vi "observacao.vi"() -> ()   [LabVIEW 2018, in "Shared_160.lvlib"] (continued)
              tunnel: [w1811 w1813] -> w1790
              tunnel: [w1811 w1814] -> w1789
              tunnel: w1788 -> [_ w1814]
              tunnel: w1787 -> [_ w1813]
              frame False {
                w1811 = 0.0 ("DeslocRA")
                n1518 = property on="Calagem" class="Bool"("Disabled"=u8 2) -> ()  [unwired: 2 in, 2 out]
              }
              frame True {
                n1519 = property on="Calagem" class="Bool"("Disabled"=u8 0) -> ()  [unwired: 2 in, 2 out]
              }
            }
            "DeslocRA" <- w1789
            "DeslocDEC" <- w1790
          }
          frame "GUIDER" {
            w1959 = 1 ("lower limit")
            w1960 = 400 ("upper limit")
            # "PROCESSO VARIABLE TRACKING"
            n1520 = Not(x="ExternalTracking") -> (.not. x?=w1945:bool)
            n1521 = call "Borda Subida.vi"("Entrada"="VARIABLE \nTRACKING") -> ("Boolean"=w1947:bool)  [unwired: 4 in]
            n1522 = call "Borda.vi"("Entrada"="VARIABLE \nTRACKING") -> ("Boolean"=w1948:bool)  [unwired: 4 in]
            n1523 = And(x=w1945, y=w1947) -> (x .and. y?=w1946:bool)
            n1524 = case shown="True" w1948 {
              frame False {
              }
              frame True {
                w2017 = "0" ("Set Point")
                w2023 = u16 2 items=["ZERO", "AH", "DEC", "TUBO", "CUP"] ("Controlador")
                w2020 = u16 1 items=["ZERO", "AH", "DEC", "TUBO", "CUP"] ("Controlador")
                # "Enviando ZERO o controlador para o movimento"
                n1525 = call "Monta Comando.vi"("Set Point"=w2017, "Comando"="GIRAR_VEL", "Dispositivo"="EIXO" ("Comando"), "Controlador"=w2020) -> ()  [unwired: 1 in, 5 out]
                n1526 = call "Monta Comando.vi"("Set Point"=w2017, "Comando"="GIRAR_VEL", "Dispositivo"="EIXO" ("Comando"), "Controlador"=w2023) -> ()  [unwired: 1 in, 5 out]
              }
            }
            n1527 = case shown="True" w1946 {
              frame False {
              }
              frame True {
                w2034 = u16 2 items=["ZERO", "AH", "DEC", "TUBO", "CUP"] ("Controlador")
                w2031 = u16 1 items=["ZERO", "AH", "DEC", "TUBO", "CUP"] ("Controlador")
                # "Enviar esses Valores \npara os controladores"
                n1528 = property on="Calagem" class="Bool"("Disabled"=u8 2) -> ()  [unwired: 2 in, 2 out]
                n1529 = Number To Decimal String(number="RA  RATE") -> (decimal integer string=w2027:string)  [unwired: 1 in]
                n1530 = Number To Decimal String(number="DEC RATE") -> (decimal integer string=w2025:string)  [unwired: 1 in]
                n1531 = call "Monta Comando.vi"("Set Point"=w2027, "Comando"="GIRAR_VEL", "Dispositivo"="EIXO" ("Comando"), "Controlador"=w2031) -> ()  [unwired: 1 in, 5 out]
                n1532 = call "Monta Comando.vi"("Set Point"=w2025, "Comando"="GIRAR_VEL", "Dispositivo"="EIXO" ("Comando"), "Controlador"=w2034) -> ()  [unwired: 1 in, 5 out]
              }
            }
            n1533 = case shown="True" "ClearDEC" {
              frame False {
              }
              frame True {
                n1534 = local write "DEC RATE"(0 ("RA  RATE")) -> ()
              }
            }
            n1535 = case shown="True" "ClearRA" {
              frame False {
              }
              frame True {
                n1536 = local write "RA  RATE"(0 ("RA  RATE")) -> ()
              }
            }
            n1537 = In Range and Coerce(upper limit=w1960, x="X STAR", lower limit=w1959) -> (In Range?=w1956:bool)  [unwired: 1 out]
            n1538 = In Range and Coerce(upper limit=w1960, x="Y STAR", lower limit=w1959) -> (In Range?=w1957:bool)  [unwired: 1 out]
            n1539 = In Range and Coerce(upper limit=w1960, x="X CENTER", lower limit=w1959) -> (In Range?=w1955:bool)  [unwired: 1 out]
            n1540 = In Range and Coerce(upper limit=w1960, x="Y CENTER", lower limit=w1959) -> (In Range?=w1954:bool)  [unwired: 1 out]
            n1541 = Compound Arithmetic op=AND(w1956, w1957, w1955, w1954, "XY CENTER") -> (w1958:bool)
            n1542 = case shown="True" w1958 {
              tunnel: "X STAR" -> [_ w1998]
              tunnel: "X CENTER" -> [_ w1997]
              tunnel: "Y STAR" -> [_ w1996]
              tunnel: "Y CENTER" -> [_ w1995]
              frame False {
              }
              frame True {
                # "MUDANÇA: IMPLEMENTADO MOV. XY DO GUIDER EM \n20-05-2011, MAS AINDA NÃO FOI TESTADO..."
                # "rad"
                # "Ativa o envio comando de deslocamento ao controlador"
                n1543 = global read "Global_Telescopio.vi" "guide_ang"() -> (w1986:string)
                n1544 = global read "Global_Telescopio.vi" "guide_nor"() -> (w1987:string)
                n1545 = global read "Global_Telescopio.vi" "guide_cas"() -> (w1994:string)
                n1546 = Subtract(x=w1998, y=w1997) -> (x-y=w1992:i32)
                n1547 = Subtract(x=w1996, y=w1995) -> (x-y=w1991:i32)
                n1548 = global read "Global_Telescopio.vi" "guide_esp"() -> (w1989:string)
                n1549 = To Double Precision Float(number=w1992) -> (double precision float=w1969:dbl)
                n1550 = To Double Precision Float(number=w1991) -> (double precision float=w1970:dbl)
                n1551 = Equal?(x=w1994, y="S") -> (x = y?=w1984:bool)
                n1552 = case shown="True" w1984 {
                  tunnel: w1987 -> [_ w2014]
                  tunnel: w1986 -> [_ w2011]
                  tunnel: [w2007 w2008] -> w1983
                  frame False {
                    # "Foco Coudé"
                    n1553 = call "AnguloFenda.vi"() -> ("AngFenda"=w2007:dbl)  [unwired: 3 in]
                  }
                  frame True {
                    # "Foco Cassegrain"
                    n1554 = Fract/Exp String To Number(use system decimal point (T)=FALSE, string=w2014) -> (number=w2009:dbl)  [unwired: 2 in, 1 out]
                    n1555 = Fract/Exp String To Number(use system decimal point (T)=FALSE, string=w2011) -> (number=w2010:dbl)  [unwired: 2 in, 1 out]
                    n1556 = Add(x=w2010, y=w2009) -> (x+y=w2008:dbl)
                  }
                }
                n1557 = Equal?(x=w1989, y="S") -> (x = y?=w1974:bool)
                n1558 = global write "Global_Telescopio.vi" "Correção Guider"("Habilita Movimento") -> ()
                n1559 = Multiply(x=0.01745329252 ("y"), y=w1983) -> (x*y=w1982:dbl)
                n1560 = Cosine(x=w1982) -> (cos(x)=w1971:dbl)
                n1561 = Sine(x=w1982) -> (sin(x)=w1972:dbl)
                n1562 = Multiply(x=w1969, y=w1971) -> (x*y=w1963:dbl)
                n1563 = Multiply(x=w1971, y=w1970) -> (x*y=w1968:dbl)
                n1564 = Multiply(x=w1970, y=w1972) -> (x*y=w1964:dbl)
                n1565 = Multiply(x=w1972, y=w1969) -> (x*y=w1967:dbl)
                n1566 = Subtract(x=w1968, y=w1967) -> (x-y=w1966:dbl)
                n1567 = Add(x=w1964, y=w1963) -> (x+y=w1965:dbl)
                n1568 = Less Than 0?(x=w1966) -> (x < 0?=w1980:bool)
                n1569 = Less Than 0?(x=w1965) -> (x < 0?=w1976:bool)
                n1570 = case shown="True" w1976 {
                  tunnel: w1974 -> [w2000 w2003]
                  tunnel: [w1999 w2004] -> w1973
                  frame False {
                    n1571 = Select(t="W" ("y"), s=w2000, f="E" ("y")) -> (s? t:f=w1999:string)
                  }
                  frame True {
                    n1572 = Select(t="E" ("y"), s=w2003, f="W" ("y")) -> (s? t:f=w2004:string)
                  }
                }
                n1573 = Select(t="S" ("y"), s=w1980, f="N" ("y")) -> (s? t:f=w1979:string)
                n1574 = Absolute Value(x=w1966) -> (abs(x)=w1977:dbl)
                n1575 = Absolute Value(x=w1965) -> (abs(x)=w1975:dbl)
                n1576 = global write "Global_Telescopio.vi" "guide_dir_we"(w1973) -> ()
                n1577 = global write "Global_Telescopio.vi" "guide_dir_ns"(w1979) -> ()
                n1578 = global write "Global_Telescopio.vi" "guide_dec"(w1977) -> ()
                n1579 = global write "Global_Telescopio.vi" "guide_asc"(w1975) -> ()
              }
            }
          }
          frame "CALIBRATION" {
            # "Alterado dia 23/07/218"
            n1580 = disable-structure shown="Disabled" {
              frame Disabled {
              }
              frame Enabled {
              }
            }
            n1581 = disable-structure shown="Disabled" {
              frame Disabled {
                w2037 = u16 4 items=["ZERO", "AH", "DEC", "TUBO", "CUP"] ("Controlador")
                n1582 = call "Monta Comando.vi"("Comando"="FECHAR", "Dispositivo"="TRAPEIRA" ("Comando"), "Controlador"=w2037) -> ()  [unwired: 2 in, 5 out]
              }
              frame Enabled {
              }
            }
            n1583 = event shown="[4] \"Coude\": Value Change" {
              selector: _ -> [_ _ _ _ _]
              dyn-events: _ -> [_ _ _ _ _]
              timeout: 10 -> [_ _ _ _ _]
              event Timeout {
                n1584 = event-data() -> ()  [unwired: 1 in, 2 out]
              }
              event "Weak": Value Change {
                w2039 = u16 15 items=["Alarme", "Atencao", "Erro", "Ocupado", "Plataforma", "LCB", "Trapeira", "Paravento", "DomoRap", "DomoCW", "DomoCCW", "TBD", "Em movimento", "TrapRUN", "TrapFCH", "TrapABT"] ("NomeStatus")
                n1585 = event-data() -> ("NewVal"=w2041:bool)  [unwired: 1 in, 5 out]
                n1586 = call "Bit Status CUP.vi"("NomeStatus"=w2039) -> ("StatBit"=w2040:bool)
                n1587 = case shown="True" w2040 {
                  tunnel: w2041 -> [w2048 _]
                  frame False {
                    w2042 = u16 4 items=["ZERO", "AH", "DEC", "TUBO", "CUP"] ("Controlador")
                    n1588 = case shown="True" w2048 {
                      tunnel: [w2049 TRUE ("WeakSel")] -> w2047
                      tunnel: [w2049 FALSE ("MediumSel")] -> w2045
                      tunnel: [0 2] -> w2044
                      tunnel: ["DESLIGAR" ("Comando") "LIGAR" ("Comando")] -> w2046
                      frame False {
                        w2049 = FALSE ("MediumSel")
                      }
                      frame True {
                        n1589 = local write "DOME"(FALSE) -> ()
                      }
                    }
                    n1590 = property on="Coude" class="Bool (strict)"("DisabledEnum"=w2044) -> ()  [unwired: 2 in, 2 out]
                    n1591 = property on="WeakSel" class="Bool (strict)"("Value"=w2047) -> ()  [unwired: 2 in, 2 out]
                    n1592 = property on="CoudeSel" class="Bool (strict)"("Value"=w2045) -> ()  [unwired: 2 in, 2 out]
                    n1593 = property on="Strong" class="Bool (strict)"("Disabled"=w2044) -> ()  [unwired: 2 in, 2 out]
                    n1594 = property on="MediumSel" class="Bool (strict)"("Value"=w2045) -> ()  [unwired: 2 in, 2 out]
                    n1595 = property on="StrongSel" class="Bool (strict)"("Value"=w2045) -> ()  [unwired: 2 in, 2 out]
                    n1596 = property on="Medium" class="Bool (strict)"("Disabled"=w2044) -> ()  [unwired: 2 in, 2 out]
                    n1597 = call "Monta Comando.vi"("Comando"=w2046, "Dispositivo"="FLAT_WEAK", "Controlador"=w2042) -> ()  [unwired: 2 in, 5 out]
                  }
                  frame True {
                    w2058 = FALSE ("Weak")
                    # "TU safe"
                    n1598 = call "Get host time.vi"() -> ("BR current time"=w2057:timestamp)  [unwired: 8 in, 3 out]
                    n1599 = Add(x=w2057, y=10.0) -> (x+y=w2061:timestamp)
                    n1600 = local write "alarm Time"(w2061) -> ()
                    n1601 = property on="Weak" class="Bool (strict)"("Value"=w2058) -> ()  [unwired: 2 in, 2 out]
                    n1602 = property on="Mensage Alarme" class="Str"("Visible"=TRUE) -> ()  [unwired: 2 in, 2 out]
                    n1603 = property on="WeakSel" class="Bool (strict)"("Value"=w2058) -> ()  [unwired: 2 in, 2 out]
                    n1604 = local write "Flag Alarm"(TRUE ("Flag Alarm")) -> ()
                  }
                }
              }
              event "Medium": Value Change {
                w2063 = u16 15 items=["Alarme", "Atencao", "Erro", "Ocupado", "Plataforma", "LCB", "Trapeira", "Paravento", "DomoRap", "DomoCW", "DomoCCW", "TBD", "Em movimento", "TrapRUN", "TrapFCH", "TrapABT"] ("NomeStatus")
                n1605 = event-data() -> ("NewVal"=w2065:bool)  [unwired: 1 in, 5 out]
                n1606 = call "Bit Status CUP.vi"("NomeStatus"=w2063) -> ("StatBit"=w2064:bool)
                n1607 = case shown="False" w2064 {
                  tunnel: w2065 -> [w2072 _]
                  frame False {
                    w2067 = u16 4 items=["ZERO", "AH", "DEC", "TUBO", "CUP"] ("Controlador")
                    n1608 = case shown="True" w2072 {
                      tunnel: [0 2] -> w2069
                      tunnel: [w2074 TRUE] -> w2070
                      tunnel: [w2074 FALSE] -> w2068
                      tunnel: ["DESLIGAR" "LIGAR"] -> w2071
                      frame False {
                        w2074 = FALSE
                      }
                      frame True {
                        n1609 = local write "DOME"(FALSE) -> ()
                      }
                    }
                    n1610 = property on="Weak" class="Bool (strict)"("Disabled"=w2069) -> ()  [unwired: 2 in, 2 out]
                    n1611 = property on="Strong" class="Bool (strict)"("Disabled"=w2069) -> ()  [unwired: 2 in, 2 out]
                    n1612 = property on="WeakSel" class="Bool (strict)"("Value"=w2068) -> ()  [unwired: 2 in, 2 out]
                    n1613 = property on="MediumSel" class="Bool (strict)"("Value"=w2070) -> ()  [unwired: 2 in, 2 out]
                    n1614 = property on="StrongSel" class="Bool (strict)"("Value"=w2068) -> ()  [unwired: 2 in, 2 out]
                    n1615 = property on="Coude" class="Bool (strict)"("DisabledEnum"=w2069) -> ()  [unwired: 2 in, 2 out]
                    n1616 = property on="CoudeSel" class="Bool (strict)"("Value"=w2068) -> ()  [unwired: 2 in, 2 out]
                    n1617 = call "Monta Comando.vi"("Comando"=w2071, "Dispositivo"="FLAT_LO", "Controlador"=w2067) -> ()  [unwired: 2 in, 5 out]
                  }
                  frame True {
                    w2082 = FALSE ("Medium")
                    # "TU safe"
                    n1618 = call "Get host time.vi"() -> ("BR current time"=w2081:timestamp)  [unwired: 8 in, 3 out]
                    n1619 = Add(x=w2081, y=10.0) -> (x+y=w2085:timestamp)
                    n1620 = local write "alarm Time"(w2085) -> ()
                    n1621 = property on="Mensage Alarme" class="Str"("Visible"=TRUE) -> ()  [unwired: 2 in, 2 out]
                    n1622 = local write "Flag Alarm"(TRUE ("Flag Alarm")) -> ()
                    n1623 = property on="Medium" class="Bool (strict)"("Value"=w2082) -> ()  [unwired: 2 in, 2 out]
                    n1624 = property on="MediumSel" class="Bool (strict)"("Value"=w2082) -> ()  [unwired: 2 in, 2 out]
                  }
                }
              }
              event "Strong": Value Change {
                w2087 = u16 15 items=["Alarme", "Atencao", "Erro", "Ocupado", "Plataforma", "LCB", "Trapeira", "Paravento", "DomoRap", "DomoCW", "DomoCCW", "TBD", "Em movimento", "TrapRUN", "TrapFCH", "TrapABT"] ("NomeStatus")
                n1625 = event-data() -> ("NewVal"=w2089:bool)  [unwired: 1 in, 5 out]
                n1626 = call "Bit Status CUP.vi"("NomeStatus"=w2087) -> ("StatBit"=w2088:bool)
                n1627 = case shown="False" w2088 {
                  tunnel: w2089 -> [w2097 _]
                  frame False {
                    w2090 = u16 4 items=["ZERO", "AH", "DEC", "TUBO", "CUP"] ("Controlador")
                    n1628 = case shown="True" w2097 {
                      tunnel: [FALSE w2104] -> w2092
                      tunnel: [w2098 w2104] -> w2096
                      tunnel: [0 2] -> w2093
                      tunnel: ["DESLIGAR" "LIGAR"] -> w2095
                      tunnel: [w2098 TRUE] -> w2094
                      frame False {
                        w2098 = FALSE
                      }
                      frame True {
                        w2104 = FALSE
                        n1629 = local write "DOME"(FALSE) -> ()
                      }
                    }
                    n1630 = property on="Medium" class="Bool (strict)"("Disabled"=w2093) -> ()  [unwired: 2 in, 2 out]
                    n1631 = property on="Weak" class="Bool (strict)"("Disabled"=w2093) -> ()  [unwired: 2 in, 2 out]
                    n1632 = property on="WeakSel" class="Bool (strict)"("Value"=w2096) -> ()  [unwired: 2 in, 2 out]
                    n1633 = property on="MediumSel" class="Bool (strict)"("Value"=w2092) -> ()  [unwired: 2 in, 2 out]
                    n1634 = property on="StrongSel" class="Bool (strict)"("Value"=w2094) -> ()  [unwired: 2 in, 2 out]
                    n1635 = property on="Coude" class="Bool (strict)"("DisabledEnum"=w2093) -> ()  [unwired: 2 in, 2 out]
                    n1636 = property on="CoudeSel" class="Bool (strict)"("Value"=w2092) -> ()  [unwired: 2 in, 2 out]
                    n1637 = call "Monta Comando.vi"("Comando"=w2095, "Dispositivo"="FLAT_HI", "Controlador"=w2090) -> ()  [unwired: 2 in, 5 out]
                  }
                  frame True {
                    w2108 = FALSE ("Strong")
                    # "TU safe"
                    n1638 = property on="StrongSel" class="Bool (strict)"("Value"=w2108) -> ()  [unwired: 2 in, 2 out]
                    n1639 = property on="Strong" class="Bool (strict)"("Value"=w2108) -> ()  [unwired: 2 in, 2 out]
                    n1640 = call "Get host time.vi"() -> ("BR current time"=w2107:timestamp)  [unwired: 8 in, 3 out]
                    n1641 = Add(x=w2107, y=10.0) -> (x+y=w2111:timestamp)
                    n1642 = local write "alarm Time"(w2111) -> ()
                    n1643 = property on="Mensage Alarme" class="Str"("Visible"=TRUE) -> ()  [unwired: 2 in, 2 out]
                    n1644 = local write "Flag Alarm"(TRUE ("Flag Alarm")) -> ()
                  }
                }
              }
              event "Coude": Value Change {
                w2113 = u16 15 items=["Alarme", "Atencao", "Erro", "Ocupado", "Plataforma", "LCB", "Trapeira", "Paravento", "DomoRap", "DomoCW", "DomoCCW", "TBD", "Em movimento", "TrapRUN", "TrapFCH", "TrapABT"] ("NomeStatus")
                n1645 = event-data() -> ("NewVal"=w2115:bool)  [unwired: 1 in, 5 out]
                n1646 = call "Bit Status CUP.vi"("NomeStatus"=w2113) -> ("StatBit"=w2114:bool)
                n1647 = case shown="False" w2114 {
                  tunnel: w2115 -> [w2122 _]
                  frame False {
                    w2116 = u16 4 items=["ZERO", "AH", "DEC", "TUBO", "CUP"] ("Controlador")
                    n1648 = case shown="True" w2122 {
                      tunnel: [FALSE w2130] -> w2119
                      tunnel: [w2124 w2130] -> w2120
                      tunnel: [0 2] -> w2118
                      tunnel: ["DESLIGAR" "LIGAR"] -> w2123
                      tunnel: [w2124 TRUE] -> w2121
                      frame False {
                        w2124 = FALSE
                      }
                      frame True {
                        w2130 = FALSE
                        n1649 = local write "DOME"(FALSE) -> ()
                      }
                    }
                    n1650 = property on="StrongSel" class="Bool (strict)"("Value"=w2120) -> ()  [unwired: 2 in, 2 out]
                    n1651 = property on="CoudeSel" class="Bool (strict)"("Value"=w2121) -> ()  [unwired: 2 in, 2 out]
                    n1652 = property on="MediumSel" class="Bool (strict)"("Value"=w2119) -> ()  [unwired: 2 in, 2 out]
                    n1653 = property on="Weak" class="Bool (strict)"("DisabledEnum"=w2118) -> ()  [unwired: 2 in, 2 out]
                    n1654 = property on="Medium" class="Bool (strict)"("DisabledEnum"=w2118) -> ()  [unwired: 2 in, 2 out]
                    n1655 = property on="Strong" class="Bool (strict)"("DisabledEnum"=w2118) -> ()  [unwired: 2 in, 2 out]
                    n1656 = property on="WeakSel" class="Bool (strict)"("Value"=w2119) -> ()  [unwired: 2 in, 2 out]
                    n1657 = call "Monta Comando.vi"("Comando"=w2123, "Dispositivo"="FLAT_COUDE", "Controlador"=w2116) -> ()  [unwired: 2 in, 5 out]
                  }
                  frame True {
                    w2134 = FALSE ("Coude")
                    # "TU safe"
                    n1658 = call "Get host time.vi"() -> ("BR current time"=w2133:timestamp)  [unwired: 8 in, 3 out]
                    n1659 = Add(x=w2133, y=10.0) -> (x+y=w2137:timestamp)
                    n1660 = local write "alarm Time"(w2137) -> ()
                    n1661 = property on="Mensage Alarme" class="Str"("Visible"=TRUE) -> ()  [unwired: 2 in, 2 out]
                    n1662 = local write "Flag Alarm"(TRUE ("Flag Alarm")) -> ()
                    n1663 = property on="CoudeSel" class="Bool (strict)"("Value"=w2134) -> ()  [unwired: 2 in, 2 out]
                    n1664 = property on="Coude" class="Bool (strict)"("Value"=w2134) -> ()  [unwired: 2 in, 2 out]
                  }
                }
              }
            }
          }
          frame "LIST" {
            n1665 = stacked-sequence {
              frame #0 {
                # "Muda nome do controle de RA para AH se MAFmax == 100"
                n1666 = case shown="True" "SET coord" {
                  frame False {
                  }
                  frame True {
                    n1667 = stacked-sequence {
                      frame #0 {
                        w2154 = "2000"
                        # "Valores aux para Detectar Edição"
                        n1668 = local read "Multicolumn Listbox"() -> (w2161:i32[])
                        n1669 = property on="Multicolumn Listbox" class="MCListbox (strict)"() -> ("Item Names"=w2159:string[][])  [unwired: 2 in, 2 out]
                        n1670 = Index Array(array=w2161, index=0) -> (element=w2158:i32)
                        n1671 = local write "FLAG SET COORD"(TRUE ("FLAG_MAG")) -> ()
                        n1672 = Index Array(array=w2159, index (row)=w2158) -> (element=w2157:string[])  [unwired: 1 in]
                        n1673 = Index Array(array=w2157, index #1=0 ("index")) -> (element #1=w2150:string, element #2=w2148:string, element #3=w2149:string, element #4=w2151:string, element #5=w2153:string, element #6=w2152:string)  [unwired: 5 in]
                        "RA AUX" <- w2148
                        "AUX EDITA Name" <- w2150
                        "AUX EDITA RA" <- w2148
                        "AUX EDITA DEC" <- w2149
                        "AUX EDITA PMRA" <- w2153
                        "AUX EDITA PMDEC" <- w2152
                        n1674 = local write "StrPointObjPMRA"(w2153) -> ()
                        n1675 = local write "StrPointObjPMDEC"(w2152) -> ()
                        n1676 = local write "StrPointObjName"(w2150) -> ()
                        n1677 = local write "StrPointObjRA"(w2148) -> ()
                        n1678 = local write "StrPointObjDEC"(w2149) -> ()
                        n1679 = local write "MAG"(w2151) -> ()
                        n1680 = local write "StrPointObjEpoch"(w2154) -> ()
                        "EPOCH AUX" <- w2154
                        "AUX EDITA EPOCH" <- w2154
                      }
                      frame #1 {
                        n1681 = case shown="False" "Case Constant\n(See Context Help) 7" {
                          frame False {
                          }
                          frame True {
                            # "Ao clicar SET COORD, fechar a aba LIST e abrir a aba POINTING"
                            n1682 = local write "Setup, Pointing & Guiding"(T2."POINTING" ("Setup, Pointing & Guiding")) -> ()
                          }
                        }
                      }
                    }
                  }
                }
                n1683 = case shown="True" "Clear ALL" {
                  frame False {
                  }
                  frame True {
                    n1684 = Two Button Dialog(message="Will you clear All Table?") -> (T button?=w2164:bool)  [unwired: 2 in]
                    n1685 = case shown="True" w2164 {
                      frame False {
                      }
                      frame True {
                        w2166 = string[][] [] ("Item Names")
                        # "Limpa a Tabela Inteira"
                        n1686 = property on="Multicolumn Listbox" class="MCListbox (strict)"("Item Names"=w2166) -> ()  [unwired: 2 in, 2 out]
                        n1687 = local write "subarray"(w2166) -> ()
                      }
                    }
                  }
                }
                n1688 = local read "MAG Max"() -> (w2140:dbl)
                n1689 = Equal?(x=100.0, y=w2140) -> (x = y?=w2139:bool)
                n1690 = case shown="False" w2139 {
                  frame False {
                    n1691 = flat-sequence {
                      frame #0 {
                        w2144 = FALSE
                        n1692 = property on="RA Max" class="DigNum (strict)"("Caption.Visible"=w2144) -> ()  [unwired: 2 in, 2 out]
                        n1693 = property on="RA Min" class="DigNum (strict)"("Caption.Visible"=w2144) -> ()  [unwired: 2 in, 2 out]
                      }
                      frame #1 {
                        w2145 = TRUE
                        n1694 = property on="RA Min" class="DigNum (strict)"("Label.Visible"=w2145) -> ()  [unwired: 2 in, 2 out]
                        n1695 = property on="RA Max" class="DigNum (strict)"("Label.Visible"=w2145) -> ()  [unwired: 2 in, 2 out]
                      }
                    }
                  }
                  frame True {
                    n1696 = flat-sequence {
                      frame #0 {
                        w2146 = FALSE
                        n1697 = property on="RA Max" class="DigNum (strict)"("Label.Visible"=w2146) -> ()  [unwired: 2 in, 2 out]
                        n1698 = property on="RA Min" class="DigNum (strict)"("Label.Visible"=w2146) -> ()  [unwired: 2 in, 2 out]
                      }
                      frame #1 {
                        w2147 = TRUE
                        n1699 = property on="RA Min" class="DigNum (strict)"("Caption.Visible"=w2147) -> ()  [unwired: 2 in, 2 out]
                        n1700 = property on="RA Max" class="DigNum (strict)"("Caption.Visible"=w2147) -> ()  [unwired: 2 in, 2 out]
                      }
                    }
                  }
                }
              }
              frame #1 {
                # "MUDANÇA:\nUPLOAD carrega\ncatálogo usuário"
                n1701 = case shown="True" "Upload" {
                  frame False {
                  }
                  frame True {
                    n1702 = File Dialog() -> (0:w2172:errorcluster, 1:w2174:bool, 3:w2173:path)  [unwired: 7 in, 1 out]
                    n1703 = Unbundle(w2172) -> ("status"=w2171:bool)  [unwired: 2 out]
                    n1704 = Not(x=w2171) -> (.not. x?=w2169:bool)
                    n1705 = And(x=w2174, y=w2169) -> (x .and. y?=w2170:bool)
                    n1706 = case shown="False" w2170 {
                      tunnel: w2173 -> [w2178 _]
                      frame False {
                        w2179 = 0 ("Slide")
                        # "Abre Arquivo Escolhido"
                        n1707 = Strip Path(path=w2178) -> (name=w2176:string)  [unwired: 1 out]
                        n1708 = Path To String(path=w2178) -> (string=w2182:string)
                        n1709 = local write "List File"(w2176) -> ()
                        n1710 = call "leexel.vi"("path"=w2182) -> ("array 5"=w2177:string[][])  [unwired: 4 in]
                        n1711 = local write "Slide"(w2179) -> ()
                        n1712 = local write "subarray"(w2177) -> ()
                        n1713 = Array Subset(array=w2177, index (row)=w2179, length (row)=10 ("length"), index (col)=w2179, length (col)=8 ("index")) -> (w2175:string[][])
                        n1714 = property on="Multicolumn Listbox" class="MCListbox (strict)"("Item Names"=w2175) -> ()  [unwired: 2 in, 2 out]
                      }
                      frame True {
                      }
                    }
                  }
                }
                n1715 = case shown="True" "Save AS" {
                  frame False {
                  }
                  frame True {
                    n1716 = File Dialog() -> (0:w2183:errorcluster, 1:w2185:bool, 3:w2184:path)  [unwired: 7 in, 1 out]
                    n1717 = Unbundle(w2183) -> ()  [unwired: 3 out]
                    n1718 = case shown="False" w2185 {
                      tunnel: w2184 -> [w2187 _]
                      frame False {
                        # "Salva Arquivo Escolhido"
                        n1719 = Path To String(path=w2187) -> (string=w2188:string)
                        n1720 = case shown="True" "Case Constant\n(See Context Help) 8" {
                          tunnel: w2188 -> [_ w2190]
                          frame False {
                          }
                          frame True {
                            n1721 = local read "subarray"() -> (w2189:string[][])
                            n1722 = call "salvaexel.vi"("appended array"=w2189, "file name p/ exell"=w2190) -> ()  [unwired: 1 in, 1 out]
                          }
                        }
                      }
                      frame True {
                      }
                    }
                  }
                }
              }
              frame #2 {
                # "Acerta Posição do Slide"
                n1723 = local read "Tot Linhas"() -> (w2196:i32)
                n1724 = Multiply(x="Slide", y=w2196) -> (x*y=w2195:dbl)
                n1725 = Divide(x=w2195, y=24.0) -> (x/y=w2193:dbl)
                n1726 = Not Equal?(x=w2193, y="Slide old") -> (x != y?=w2198:bool)
                n1727 = case shown="True" w2198 {
                  tunnel: w2193 -> [_ w2203]
                  frame False {
                  }
                  frame True {
                    n1728 = stacked-sequence {
                      seq-local: [w2207 _] -> [_ w2212]
                      tunnel: w2203 -> [w2208 _]
                      frame #0 {
                        # "Previne estouro\nda planilha"
                        n1729 = local read "Tot Linhas"() -> (w2206:i32)
                        n1730 = Subtract(x=w2206, y=10) -> (x-y=w2204:i32)
                        n1731 = Greater Or Equal?(x=w2208, y=w2204) -> (x >= y?=w2209:bool)
                        n1732 = case shown="False" w2209 {
                          tunnel: [w2210 w2211] -> w2207
                          tunnel: w2204 -> [_ w2211]
                          tunnel: w2208 -> [w2210 _]
                          frame False {
                          }
                          frame True {
                          }
                        }
                      }
                      frame #1 {
                        n1733 = local read "subarray"() -> (w2214:string[][])
                        n1734 = Array Subset(array=w2214, index (row)=w2212, length (row)=11 ("length"), index (col)=0 ("index"), length (col)=8 ("index")) -> (w2213:string[][])
                        n1735 = property on="Multicolumn Listbox" class="MCListbox (strict)"("Item Names"=w2213) -> ()  [unwired: 2 in, 2 out]
                        n1736 = local write "Slide old"(w2212) -> ()
                      }
                    }
                  }
                }
                n1737 = case shown="True" "Open BSC" {
                  frame False {
                  }
                  frame True {
                    n1738 = stacked-sequence {
                      frame #0 {
                        w2251 = FALSE
                        # "MUDANÇA:\nUPLOAD carrega\ncatálogo usuário"
                        # "Faz Aparecer os Botões"
                        n1739 = property on="Delete" class="Bool"("Visible"=w2251) -> ()  [unwired: 2 in, 2 out]
                        n1740 = property on="EDIT" class="Bool"("Visible"=w2251) -> ()  [unwired: 2 in, 2 out]
                        n1741 = property on="Clear ALL" class="Bool"("Visible"=w2251) -> ()  [unwired: 2 in, 2 out]
                        n1742 = property on="Save AS" class="Bool"("Visible"=w2251) -> ()  [unwired: 2 in, 2 out]
                        n1743 = property on="Save" class="Bool"("Visible"=w2251) -> ()  [unwired: 2 in, 2 out]
                        n1744 = property on="Insert" class="Bool"("Visible"=w2251) -> ()  [unwired: 2 in, 2 out]
                        n1745 = property on="Upload" class="Bool"("Visible"=TRUE) -> ()  [unwired: 2 in, 2 out]
                      }
                      frame #1 {
                        w2252 = "C:\\TCS\\ARQUIVOS\\BSC_08.txt"
                        w2259 = 0 ("Slide")
                        # "Cria e Lê arquivo\nonde voce está\ntrabalhando"
                        n1746 = local write "Slide"(w2259) -> ()
                        n1747 = call "leexel.vi"("path"=w2252) -> ("array 5"=w2257:string[][])  [unwired: 4 in]
                        "subarray" <- w2257
                        n1748 = Array Subset(array=w2257, index (row)=w2259, length (row)=11 ("length"), index (col)=w2259, length (col)=8 ("index")) -> (w2260:string[][])
                        n1749 = Array Size(array=w2257) -> (size(s)=w2258:i32[])
                        n1750 = String To Path(string=w2252) -> (path=w2254:path)
                        n1751 = property on="Multicolumn Listbox" class="MCListbox (strict)"("Item Names"=w2260) -> ()  [unwired: 2 in, 2 out]
                        n1752 = Strip Path(path=w2254) -> (name=→"List File":string)  [unwired: 1 out]
                        n1753 = Index Array(array=w2258, index=0) -> (element=→"Tot Linhas":i32)
                        "Saida Path string" <- w2252
                      }
                      frame #2 {
                        n1754 = local read "Tot Linhas"() -> (w2271:i32)
                        n1755 = Quotient & Remainder(x=10000, y=w2271) -> (floor(x/y)=w2269:i32)  [unwired: 1 out]
                        n1756 = Divide(x=w2269, y=1000) -> (x/y=w2266:dbl)
                        n1757 = Multiply(x=w2266, y=24.0) -> (x*y=w2267:dbl)
                        n1758 = property on="Slide" class="Slide (strict)"("Data Entry Limits:Increment"=w2267) -> ()  [unwired: 2 in, 2 out]
                        "ScaleMax" <- "24" ("ScaleMax")
                        "ScaleMin" <- "0" ("ScaleMin")
                      }
                    }
                  }
                }
                n1759 = case shown="True" "Save" {
                  frame False {
                  }
                  frame True {
                    w2246 = "C:\\TCS\\ARQUIVOS\\List.lst"
                    # "Cria e Lê arquivo\nonde voce está\ntrabalhando"
                    n1760 = String To Path(string=w2246) -> (path=w2245:path)
                    n1761 = stacked-sequence {
                      tunnel: w2245 -> [w2247 _]
                      tunnel: w2246 -> [_ w2249]
                      frame #0 {
                        # "Apaga o arquivo"
                        n1762 = Delete(path (use dialog)=w2247) -> ()  [unwired: 4 in, 3 out]
                      }
                      frame #1 {
                        # "Salva a lista"
                        n1763 = local read "subarray"() -> (w2248:string[][])
                        n1764 = call "salvaexel.vi"("appended array"=w2248, "file name p/ exell"=w2249) -> ()  [unwired: 1 in, 1 out]
                      }
                    }
                  }
                }
                n1765 = case shown="True" "Delete" {
                  frame False {
                  }
                  frame True {
                    n1766 = local read "Multicolumn Listbox"() -> (w2224:i32[])
                    n1767 = Index Array(array=w2224, index=0) -> (element=w2218:i32)
                    n1768 = Number To Decimal String(number=w2218) -> (decimal integer string=w2221:string)  [unwired: 1 in]
                    n1769 = Concatenate Strings("Delete Line Number: " ("string"), w2221) -> (w2219:string)
                    n1770 = Two Button Dialog(message=w2219) -> (T button?=w2220:bool)  [unwired: 2 in]
                    n1771 = case shown="True" w2220 {
                      tunnel: w2218 -> [_ w2225]
                      frame False {
                      }
                      frame True {
                        n1772 = stacked-sequence {
                          tunnel: w2225 -> [w2229 _]
                          frame #0 {
                            # "Apaga a Coluna Escolhida"
                            n1773 = property on="Multicolumn Listbox" class="MCListbox (strict)"() -> ("Item Names"=w2232:string[][])  [unwired: 2 in, 2 out]
                            n1774 = local read "Slide"() -> (w2230:dbl)
                            n1775 = local read "subarray"() -> (w2227:string[][])
                            n1776 = Add(x=w2229, y=w2230) -> (x+y=w2228:dbl)
                            n1777 = Delete From Array(array=w2232, index (row)=w2229) -> (array with subset deleted=w2231:string[][])  [unwired: 2 in, 1 out]
                            n1778 = Delete From Array(array=w2227, index (row)=w2228) -> (array with subset deleted=w2226:string[][])  [unwired: 2 in, 1 out]
                            n1779 = local write "subarray"(w2226) -> ()
                            n1780 = property on="Multicolumn Listbox" class="MCListbox (strict)"("Item Names"=w2231) -> ()  [unwired: 2 in, 2 out]
                          }
                          frame #1 {
                            # "Volta para a coluna Zero"
                            n1781 = local write "Multicolumn Listbox"(i32[] [0] ("Multicolumn Listbox")) -> ()
                          }
                        }
                      }
                    }
                  }
                }
                n1782 = case shown="True" "Insert" {
                  frame False {
                  }
                  frame True {
                    n1783 = stacked-sequence {
                      seq-local: [w2235 _ _] -> [_ w2237 _]
                      seq-local: [w2234 _ _] -> [_ w2236 _]
                      frame #0 {
                        n1784 = call "Tela_Set_Coordenadas.vi"() -> ("Saída"=w2235:bool, "Val Saída"=w2234:string[])  [unwired: 4 in]
                      }
                      frame #1 {
                        n1785 = case shown="True" w2237 {
                          tunnel: w2236 -> [_ w2238]
                          frame False {
                          }
                          frame True {
                            # "Insere Linha Preenchida"
                            n1786 = local read "subarray"() -> (w2240:string[][])
                            n1787 = property on="Multicolumn Listbox" class="MCListbox (strict)"() -> ("Item Names"=w2242:string[][])  [unwired: 2 in, 2 out]
                            n1788 = Build Array (concatenate)(w2242, w2238) -> (w2241:string[][])
                            n1789 = Build Array (concatenate)(w2240, w2238) -> (w2239:string[][])
                            n1790 = property on="Multicolumn Listbox" class="MCListbox (strict)"("Item Names"=w2241) -> ()  [unwired: 2 in, 2 out]
                            n1791 = local write "subarray"(w2239) -> ()
                          }
                        }
                      }
                      frame #2 {
                        # "Depois de inserir um novo objeto na tabela,\n com o comando INSERT, mudar o objeto \nselecionado para esse novo registro."
                        n1792 = property on="Multicolumn Listbox" class="MCListbox (strict)"() -> ("Number of Rows"=w2244:u32)  [unwired: 2 in, 2 out]
                        n1793 = Build Array(w2244) -> (w2243:u32[])
                        n1794 = local write "Multicolumn Listbox"(w2243) -> ()
                      }
                    }
                  }
                }
                n1795 = property on="Multicolumn Listbox" class="MCListbox (strict)"("Selection Color"=u32 10336195) -> ()  [unwired: 2 in, 2 out]
              }
              frame #3 {
                # "Editar a Lista"
                n1796 = case shown="True" "EDIT" {
                  frame False {
                  }
                  frame True {
                    (unwired) "Edit the marked Line and soon after presses SAVE"
                    n1797 = call "Edita_lista.vi"() -> ("lista Auxiliar"=w2294:string[][])  [unwired: 5 in]
                    n1798 = property on="Multicolumn Listbox" class="MCListbox (strict)"("Item Names"=w2294) -> ()  [unwired: 2 in, 2 out]
                  }
                }
                n1799 = case shown="True" "Open" {
                  frame False {
                  }
                  frame True {
                    n1800 = stacked-sequence {
                      frame #0 {
                        w2274 = TRUE
                        # "Faz Aparecer os Botões"
                        n1801 = property on="Delete" class="Bool"("Visible"=w2274) -> ()  [unwired: 2 in, 2 out]
                        n1802 = property on="EDIT" class="Bool"("Visible"=w2274) -> ()  [unwired: 2 in, 2 out]
                        n1803 = property on="Clear ALL" class="Bool"("Visible"=w2274) -> ()  [unwired: 2 in, 2 out]
                        n1804 = property on="Upload" class="Bool"("Visible"=w2274) -> ()  [unwired: 2 in, 2 out]
                        n1805 = property on="Save AS" class="Bool"("Visible"=w2274) -> ()  [unwired: 2 in, 2 out]
                        n1806 = property on="Save" class="Bool"("Visible"=w2274) -> ()  [unwired: 2 in, 2 out]
                        n1807 = property on="Insert" class="Bool"("Visible"=w2274) -> ()  [unwired: 2 in, 2 out]
                      }
                      frame #1 {
                        w2282 = 0 ("Slide")
                        w2278 = "C:\\TCS\\ARQUIVOS\\List.lst"
                        n1808 = String To Path(string=w2278) -> (path=w2285:path)
                        n1809 = local write "Saida Path string"(w2278) -> ()
                        n1810 = call "leexel.vi"("path"=w2278) -> ("array 5"=w2277:string[][])  [unwired: 4 in]
                        n1811 = Strip Path(path=w2285) -> (name=w2284:string)  [unwired: 1 out]
                        n1812 = local write "List File"(w2284) -> ()
                        n1813 = local write "subarray"(w2277) -> ()
                        n1814 = Array Subset(array=w2277, index (row)=w2282, length (row)=10 ("length"), index (col)=w2282, length (col)=8 ("index")) -> (w2281:string[][])
                        n1815 = local write "Slide"(w2282) -> ()
                        n1816 = Array Size(array=w2277) -> (size(s)=w2275:i32[])
                        n1817 = property on="Multicolumn Listbox" class="MCListbox (strict)"("Item Names"=w2281) -> ()  [unwired: 2 in, 2 out]
                        n1818 = Index Array(array=w2275, index=0) -> (element=w2276:i32)
                        n1819 = local write "Tot Linhas"(w2276) -> ()
                      }
                      frame #2 {
                        w2286 = ""
                        n1820 = local read "Tot Linhas"() -> (w2293:i32)
                        n1821 = Quotient & Remainder(x=10000, y=w2293) -> (floor(x/y)=w2291:i32)  [unwired: 1 out]
                        n1822 = Divide(x=w2291, y=1000) -> (x/y=w2288:dbl)
                        n1823 = Multiply(x=w2288, y=24.0) -> (x*y=w2289:dbl)
                        n1824 = property on="Slide" class="Slide (strict)"("Data Entry Limits:Increment"=w2289) -> ()  [unwired: 2 in, 2 out]
                        n1825 = local write "ScaleMin"(w2286) -> ()
                        n1826 = local write "ScaleMax"(w2286) -> ()
                      }
                    }
                  }
                }
              }
              frame #4 {
                n1827 = case shown="True" "Filter RA" {
                  frame False {
                  }
                  frame True {
                    n1828 = while {
                      shift-right: [w2297] -> _
                      shift-left: "inicio" -> [w2299]
                      stop <- w2298 stop-if-true
                      n1829 = case shown="\"filtra\"" w2299 {
                        tunnel: [FALSE w2349 TRUE TRUE] -> w2298
                        tunnel: [w2319 w2350 "fim" "fim"] -> w2297
                        frame "inicio" {
                          # "RAmin"
                          # "RAmax"
                          # "Testa se:\n| Ramax - Ramin | >=1\n|Decmax -Decmin | >=1\n|Magmax -Magmin | >=1"
                          n1830 = local read "MAG Max"() -> (w2313:dbl)
                          n1831 = local read "MAG Min"() -> (w2328:dbl)
                          n1832 = Equal?(x=100.0, y=w2313) -> (x = y?=w2305:bool)
                          n1833 = Subtract(x=w2313, y=w2328) -> (x-y=w2325:dbl)
                          n1834 = case shown="True" w2305 {
                            tunnel: "RA Min" -> [w2333 w2341]
                            tunnel: [w2333 w2340] -> w2300
                            tunnel: "RA Max" -> [w2332 w2342]
                            tunnel: [w2332 w2337] -> w2301
                            frame False {
                            }
                            frame True {
                              w2346 = 24 ("RA Max")
                              # "12h/PI()"
                              # "TS, rad"
                              # "TS, hora"
                              # "RAmin"
                              # "RAmax"
                              # "AHmax"
                              # "AHmin"
                              # "MUDANÇA 7/4/2011:\nSe MAGmax >= 100,\ntratar RA como AH."
                              n1835 = global read "Global_Telescopio.vi" "Sideral Time"() -> (w2336:dbl)
                              n1836 = Multiply(x=w2336, y=3.8197) -> (x*y=w2335:dbl)
                              n1837 = To Long Integer(number=w2335) -> (32bit integer=w2343:i32)
                              n1838 = Subtract(x=w2343, y=w2342) -> (x-y=w2339:i32)
                              n1839 = Subtract(x=w2343, y=w2341) -> (x-y=w2338:i32)
                              n1840 = Add(x=w2346, y=w2339) -> (x+y=w2345:i32)
                              n1841 = Less Than 0?(x=w2339) -> (x < 0?=w2348:bool)
                              n1842 = Add(x=w2346, y=w2338) -> (x+y=w2344:i32)
                              n1843 = Less Than 0?(x=w2338) -> (x < 0?=w2347:bool)
                              n1844 = Select(t=w2345, s=w2348, f=w2339) -> (s? t:f=w2340:i32)
                              n1845 = Select(t=w2344, s=w2347, f=w2338) -> (s? t:f=w2337:i32)
                            }
                          }
                          n1846 = Less?(x=w2325, y=1.0) -> (x < y?=w2322:bool)
                          n1847 = local read "DEC Max"() -> (w2330:i32)
                          n1848 = local read "DEC Min"() -> (w2329:i32)
                          n1849 = local write "RA Min 2"(w2300) -> ()
                          n1850 = local write "RA Max 2"(w2301) -> ()
                          n1851 = Less?(x=w2301, y=w2300) -> (x < y?=w2306:bool)
                          "FiltroDuplo" <- w2306
                          n1852 = Equal?(x=w2301, y=w2300) -> (x = y?=w2304:bool)
                          n1853 = Add(x=w2301, y=24 ("RA Max")) -> (x+y=w2310:i32)
                          n1854 = Subtract(x=w2310, y=w2300) -> (x-y=w2309:i32)
                          n1855 = Subtract(x=w2330, y=w2329) -> (x-y=w2327:i32)
                          n1856 = Greater?(x=w2309, y=12) -> (0:w2307:bool)
                          n1857 = control-ref of="Erro"() -> (w2316:refnum<vi>)
                          n1858 = Less?(x=w2327, y=1) -> (x < y?=w2323:bool)
                          n1859 = And(x=w2307, y=w2306) -> (x .and. y?=w2314:bool)
                          n1860 = property class="Bool (strict)"(reference=w2316, "Boolean Text.Text"="WAIT") -> ()  [unwired: 1 in, 2 out]
                          n1861 = Compound Arithmetic op=OR(w2314, w2304, w2323, w2322) -> (w2321:bool)
                          n1862 = Select(t="erro", s=w2321, f="filtra") -> (s? t:f=w2319:string)
                          "Erro" <- FALSE ("Fim")
                        }
                        frame "filtra" {
                          n1863 = stacked-sequence {
                            seq-local: [w2354 _ _ _] -> [_ w2397 _ _]
                            seq-local: [_ w2398 _ _] -> [_ _ w2417 _]
                            seq-local: [_ _ w2418 _] -> [_ _ _ w2443]
                            tunnel: [_ _ _ "fim"] -> w2350
                            tunnel: [_ _ _ FALSE] -> w2349
                            frame #0 {
                              n1864 = property on="EDIT" class="Bool"() -> ("Visible"=w2351:bool)  [unwired: 2 in, 2 out]
                              n1865 = case shown="True" w2351 {
                                tunnel: ["C:\\TCS\\ARQUIVOS\\BSC_08.txt" "C:\\TCS\\ARQUIVOS\\List.lst"] -> w2353
                                frame False {
                                }
                                frame True {
                                }
                              }
                              n1866 = call "leexel.vi"("path"=w2353) -> ("array 5"=w2352:string[][])  [unwired: 4 in]
                              n1867 = Index Array(array=w2352, index (col)=1 ("disabled index (col)")) -> (element=w2356:string[])  [unwired: 1 in]
                              n1868 = for {
                                tunnel: w2356 -> [w2372] mode=indexing
                                shift-right: [w2366] -> w2354
                                shift-left: string[][] [] ("Item Names") -> [w2368]
                                tunnel: w2352 -> [w2365] mode=indexing
                                # "Filtro de RA"
                                n1869 = local read "FiltroDuplo"() -> (w2364:bool)
                                n1870 = String Subset(string=w2372, offset (0)=0, length (rest)=2 ("length (rest)")) -> (substring=w2369:string)
                                n1871 = Decimal String To Number(string=w2369) -> (number=w2363:i32)  [unwired: 2 in, 1 out]
                                n1872 = case shown="False" w2364 {
                                tunnel: "RA Max 2" -> [w2377 w2382]
                                tunnel: "RA Min 2" -> [w2376 w2379]
                                tunnel: [w2375 w2384] -> w2367
                                tunnel: w2363 -> [w2374 w2383]
                                tunnel: [FALSE w2378] -> w2362
                                frame False {
                                n1873 = In Range and Coerce(upper limit=w2377, x=w2374, lower limit=w2376) -> (In Range?=w2375:bool)  [unwired: 1 out]
                                }
                                frame True {
                                n1874 = In Range and Coerce(upper limit=w2382, x=w2383, lower limit=0 ("upper limit")) -> (In Range?=w2385:bool)  [unwired: 1 out]
                                n1875 = In Range and Coerce(upper limit=24 ("lower limit"), x=w2383, lower limit=w2379) -> (In Range?=w2378:bool)  [unwired: 1 out]
                                n1876 = Or(x=w2385, y=w2378) -> (x .or. y?=w2384:bool)
                                }
                                }
                                n1877 = case shown="True" w2367 {
                                tunnel: w2368 -> [w2386 w2390]
                                tunnel: [w2386 w2389] -> w2366
                                tunnel: w2365 -> [_ w2388]
                                tunnel: w2362 -> [_ w2387]
                                frame False {
                                }
                                frame True {
                                n1878 = case shown="False" w2387 {
                                tunnel: w2390 -> [w2393 w2395]
                                tunnel: [w2392 w2394] -> w2389
                                tunnel: w2388 -> [w2391 w2396]
                                frame False {
                                n1879 = Build Array (concatenate)(w2393, w2391) -> (w2392:string[][])
                                }
                                frame True {
                                n1880 = Build Array (concatenate)(w2396, w2395) -> (w2394:string[][])
                                }
                                }
                                }
                                }
                              }
                            }
                            frame #1 {
                              # "Filtro de DEC"
                              n1881 = Index Array(array=w2397, index (col)=2 ("disabled index (col)")) -> (element=w2400:string[])  [unwired: 1 in]
                              n1882 = for {
                                tunnel: w2400 -> [w2412] mode=indexing
                                shift-right: [w2405] -> w2398
                                shift-left: string[][] [] ("Item Names") -> [w2407]
                                tunnel: w2397 -> [w2404] mode=indexing
                                n1883 = String Subset(string=w2412, offset (0)=0, length (rest)=3 ("length (rest)")) -> (substring=w2409:string)
                                n1884 = Decimal String To Number(string=w2409) -> (number=w2408:i32)  [unwired: 2 in, 1 out]
                                n1885 = In Range and Coerce(upper limit="DEC Max", x=w2408, lower limit="DEC Min") -> (In Range?=w2406:bool)  [unwired: 1 out]
                                n1886 = case shown="True" w2406 {
                                tunnel: w2407 -> [w2413 w2416]
                                tunnel: [w2413 w2415] -> w2405
                                tunnel: w2404 -> [_ w2414]
                                frame False {
                                }
                                frame True {
                                n1887 = Build Array (concatenate)(w2416, w2414) -> (w2415:string[][])
                                }
                                }
                              }
                            }
                            frame #2 {
                              # "Filtro de MAG"
                              n1888 = Index Array(array=w2417, index (col)=3 ("disabled index (col)")) -> (element=w2420:string[])  [unwired: 1 in]
                              n1889 = for {
                                tunnel: w2420 -> [w2422] mode=indexing
                                shift-right: [w2426] -> w2418
                                shift-left: string[][] [] ("Item Names") -> [w2430]
                                tunnel: w2417 -> [w2428] mode=indexing
                                n1890 = Fract/Exp String To Number(use system decimal point (T)=FALSE, string=w2422) -> (number=w2425:dbl)  [unwired: 2 in, 1 out]
                                n1891 = In Range and Coerce(upper limit="MAG Max", x=w2425, lower limit="MAG Min") -> (In Range?=w2429:bool)  [unwired: 1 out]
                                n1892 = case shown="True" w2429 {
                                tunnel: w2430 -> [w2431 w2434]
                                tunnel: [w2431 w2433] -> w2426
                                tunnel: w2428 -> [_ w2432]
                                frame False {
                                }
                                frame True {
                                n1893 = Build Array (concatenate)(w2434, w2432) -> (w2433:string[][])
                                }
                                }
                              }
                            }
                            frame #3 {
                              w2435 = 0 ("index")
                              n1894 = local write "subarray"(w2443) -> ()
                              n1895 = Array Size(array=w2443) -> (size(s)=w2455:i32[])
                              n1896 = Index Array(array=w2455, index=0) -> (element=w2448:i32)
                              n1897 = local write "Tot Linhas"(w2448) -> ()
                              n1898 = local write "Slide old"(w2435) -> ()
                              n1899 = local write "Slide"(w2435) -> ()
                              n1900 = Array Subset(array=w2443, index (row)=w2435, length (row)=11 ("length"), index (col)=0 ("index"), length (col)=8 ("index")) -> (w2444:string[][])
                              n1901 = property on="Multicolumn Listbox" class="MCListbox (strict)"("Item Names"=w2444) -> ()  [unwired: 2 in, 2 out]
                              n1902 = Quotient & Remainder(x=10000, y=w2448) -> (floor(x/y)=w2452:i32)  [unwired: 1 out]
                              n1903 = Divide(x=w2452, y=1000) -> (x/y=w2450:dbl)
                              n1904 = control-ref of="Erro"() -> (w2439:refnum<vi>)
                              n1905 = Multiply(x=w2450, y=24.0) -> (x*y=w2437:dbl)
                              n1906 = property class="Bool (strict)"(reference=w2439, "Boolean Text.Text"="") -> ()  [unwired: 1 in, 2 out]
                              n1907 = Decrement(x=w2437) -> (x-1=w2436:dbl)
                              n1908 = property on="Slide" class="Slide (strict)"("Data Entry Limits:Increment"=w2436) -> ()  [unwired: 2 in, 2 out]
                              n1909 = local write "Erro"(FALSE ("Erro")) -> ()
                            }
                          }
                        }
                        frame "erro", Default {
                          n1910 = control-ref of="Erro"() -> (w2457:refnum<vi>)
                          n1911 = property class="Bool (strict)"(reference=w2457, "Boolean Text.Text"="ERROR") -> ()  [unwired: 1 in, 2 out]
                          n1912 = local write "Erro"(TRUE ("Erro")) -> ()
                        }
                        frame "fim" {
                          n1913 = local read "RA Max 2"() -> (w2462:i32)
                          n1914 = local read "RA Min 2"() -> (w2461:i32)
                          n1915 = Number To Decimal String(number=w2461) -> (decimal integer string=w2464:string)  [unwired: 1 in]
                          n1916 = Number To Decimal String(number=w2462) -> (decimal integer string=w2463:string)  [unwired: 1 in]
                          n1917 = local write "ScaleMin"(w2464) -> ()
                          n1918 = local write "ScaleMax"(w2463) -> ()
                        }
                      }
                    }
                  }
                }
              }
            }
          }
          frame " INSTRUMENT " {
            n1919 = case shown="\"Coude\", Default" "TabInstrumento" {
              frame "Casseg." {
                w2478 = u16 13 items=["Alarme", "Atencao", "Erro", "Ocupado", "PosSecund", "PosConj#3", "MovFoco", "MovCjto#3", "Mov#4", "Mov#3", "Mov#2", "EspLamp", "HE", "NE", "EspLampRepouso", "EspLampCalibra"] ("NomeStatus")
                w2477 = u16 12 items=["Alarme", "Atencao", "Erro", "Ocupado", "PosSecund", "PosConj#3", "MovFoco", "MovCjto#3", "Mov#4", "Mov#3", "Mov#2", "EspLamp", "HE", "NE", "EspLampRepouso", "EspLampCalibra"] ("NomeStatus")
